vi "topStack.vi"(8 "error in (no error)":errorcluster, 9 "pilha input":T1[](array[typedef]), 11 "Utilities in":refnum<class "Utilities.lvclass">) -> (0 "error out":errorcluster, 1 "top":T1, 3 "Utilities out":refnum<class "Utilities.lvclass">)   [LabVIEW 2018, in "Utilities.lvclass"]
uses:
  Utilities.lvclass
  sslview/Util/segment.ctl
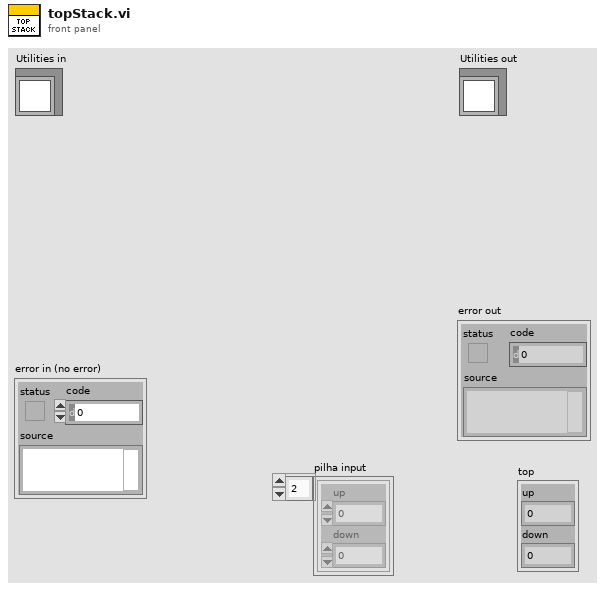
[diagram p1: front panel]
types:
  T1 = typedef "segment.ctl" = cluster{"up":dbl, "down":dbl}
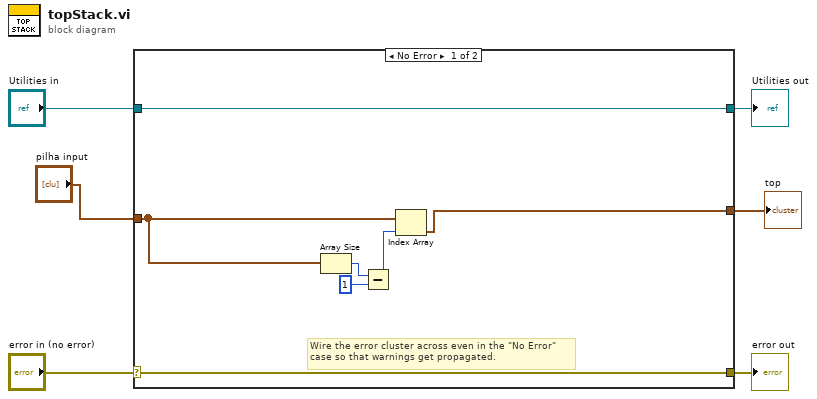
[diagram p0: block diagram]
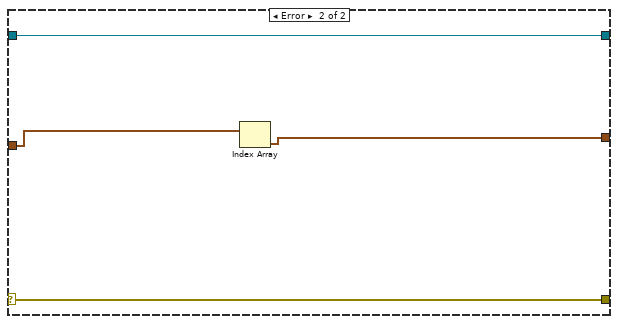
[diagram p2: hidden frame]
diagram:
  n1 = case shown="No Error" "error in (no error)" {
    selector: "error in (no error)" -> [w12 w17]
    tunnel: [w12 w17] -> w5
    tunnel: [w13 w16] -> w3
    tunnel: "Utilities in" -> [w13 w16]
    tunnel: "pilha input" -> [w8 w15]
    tunnel: [w7 w14] -> w1
    frame No Error {
      # "Wire the error cluster across even in the \"No Error\"\ncase so that warnings get propagated."
      n2 = Array Size(array=w8) -> (size(s)=w11:i32)
      n3 = Subtract(x=w11, y=1) -> (x-y=w9:i32)
      n4 = Index Array(array=w8, index=w9) -> (element=w7:T1)
    }
    frame Error {
      n5 = Index Array(array=w15) -> (element=w14:T1)  [unwired: 1 in]
    }
  }
  "error out" <- w5
  "Utilities out" <- w3
  "top" <- w1
